vi "Header data_Cnsl.vi"(0 "base path":path=path "C:/", 5 "prompt (Create Folder)":string="logsConsole", 7 "file name":string, 11 "Error In":errorcluster) -> (4 "refnum out":refnum<file>, 15 "error out":errorcluster)   [LabVIEW 2018]
uses:
  Global_usbComm.vi
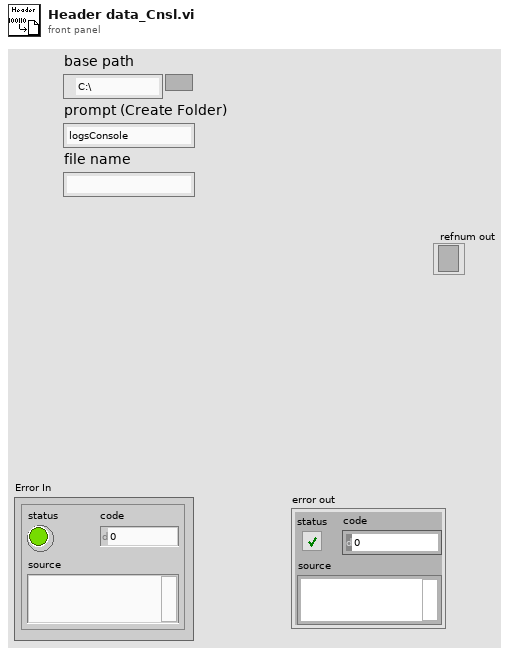
[diagram p1: front panel]
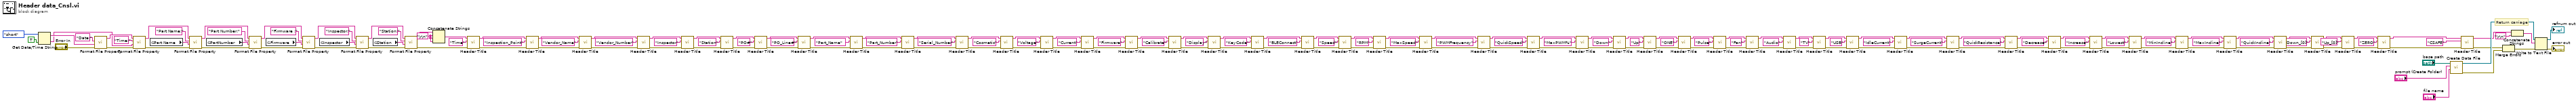
[diagram p0: block diagram]
diagram:
  w38 = "\r\n"
  # "Return carriage"
  n1 = Get Date/Time String(date format (0)=enum16{"short", "long", "abbreviated"}."short", want seconds? (F)=TRUE) -> (date string=w49:string, time string=w48:string)  [unwired: 1 in]
  n2 = call "Format File Property.vi"("Error In"="Error In", "File Property Value"=w49, "File Property Name"="Date:") -> ("Error Out"=w180:errorcluster, "String out"=w124:string)  [unwired: 7 in]
  n3 = call "Format File Property.vi"("Error In"=w180, "File Property Value"=w48, "File Property Name"="Time:", "String in"=w124) -> ("Error Out"=w41:errorcluster, "String out"=w42:string)  [unwired: 6 in]
  n4 = global read "Global_usbComm.vi" "Part Name"() -> (w112:string)
  n5 = call "Format File Property.vi"("Error In"=w41, "File Property Value"=w112, "File Property Name"="Part Name:", "String in"=w42) -> ("Error Out"=w175:errorcluster, "String out"=w122:string)  [unwired: 6 in]
  n6 = global read "Global_usbComm.vi" "PartNumber"() -> (w111:string)
  n7 = call "Format File Property.vi"("Error In"=w175, "File Property Value"=w111, "File Property Name"="Part Number:", "String in"=w122) -> ("Error Out"=w181:errorcluster, "String out"=w121:string)  [unwired: 6 in]
  n8 = global read "Global_usbComm.vi" "Firmware"() -> (w110:string)
  n9 = call "Format File Property.vi"("Error In"=w181, "File Property Value"=w110, "File Property Name"="Firmware :", "String in"=w121) -> ("Error Out"=w36:errorcluster, "String out"=w37:string)  [unwired: 6 in]
  n10 = global read "Global_usbComm.vi" "Inspector"() -> (w34:string)
  n11 = call "Format File Property.vi"("Error In"=w36, "File Property Value"=w34, "File Property Name"="Inspector:", "String in"=w37) -> ("Error Out"=w179:errorcluster, "String out"=w123:string)  [unwired: 6 in]
  n12 = global read "Global_usbComm.vi" "Station"() -> (w33:string)
  n13 = call "Format File Property.vi"("Error In"=w179, "File Property Value"=w33, "File Property Name"="Station:", "String in"=w123) -> ("Error Out"=w6:errorcluster, "String out"=w35:string)  [unwired: 6 in]
  n14 = Concatenate Strings(w35, w38, w38, w38) -> (w7:string)
  n15 = call "Header Title.vi"("Error In"=w6, "Header Title"="Time", "String in"=w7) -> ("Error Out"=w3:errorcluster, "String out"=w2:string)  [unwired: 7 in]
  n16 = call "Header Title.vi"("Error In"=w3, "Header Title"="Inspection_Point", "String in"=w2) -> ("Error Out"=w4:errorcluster, "String out"=w5:string)  [unwired: 7 in]
  n17 = call "Header Title.vi"("Error In"=w4, "Header Title"="Vendor_Name" ("File Property Name"), "String in"=w5) -> ("Error Out"=w23:errorcluster, "String out"=w31:string)  [unwired: 7 in]
  n18 = call "Header Title.vi"("Error In"=w23, "Header Title"="Vendor_Number" ("File Property Name"), "String in"=w31) -> ("Error Out"=w22:errorcluster, "String out"=w24:string)  [unwired: 7 in]
  n19 = call "Header Title.vi"("Error In"=w22, "Header Title"="Inspector" ("File Property Name"), "String in"=w24) -> ("Error Out"=w21:errorcluster, "String out"=w27:string)  [unwired: 7 in]
  n20 = call "Header Title.vi"("Error In"=w21, "Header Title"="Station" ("File Property Name"), "String in"=w27) -> ("Error Out"=w20:errorcluster, "String out"=w26:string)  [unwired: 7 in]
  n21 = call "Header Title.vi"("Error In"=w20, "Header Title"="PO#" ("File Property Name"), "String in"=w26) -> ("Error Out"=w14:errorcluster, "String out"=w13:string)  [unwired: 7 in]
  n22 = call "Header Title.vi"("Error In"=w14, "Header Title"="PO_Line#", "String in"=w13) -> ("Error Out"=w11:errorcluster, "String out"=w12:string)  [unwired: 7 in]
  n23 = call "Header Title.vi"("Error In"=w11, "Header Title"="Part_Name" ("File Property Name"), "String in"=w12) -> ("Error Out"=w16:errorcluster, "String out"=w18:string)  [unwired: 7 in]
  n24 = call "Header Title.vi"("Error In"=w16, "Header Title"="Part_Number" ("File Property Name"), "String in"=w18) -> ("Error Out"=w9:errorcluster, "String out"=w8:string)  [unwired: 7 in]
  n25 = call "Header Title.vi"("Error In"=w9, "Header Title"="Serial_Number" ("string"), "String in"=w8) -> ("Error Out"=w128:errorcluster, "String out"=w127:string)  [unwired: 7 in]
  n26 = call "Header Title.vi"("Error In"=w128, "Header Title"="Cosmetic", "String in"=w127) -> ("Error Out"=w132:errorcluster, "String out"=w131:string)  [unwired: 7 in]
  n27 = call "Header Title.vi"("Error In"=w132, "Header Title"="Voltage", "String in"=w131) -> ("Error Out"=w125:errorcluster, "String out"=w126:string)  [unwired: 7 in]
  n28 = call "Header Title.vi"("Error In"=w125, "Header Title"="Current" ("string"), "String in"=w126) -> ("Error Out"=w94:errorcluster, "String out"=w95:string)  [unwired: 7 in]
  n29 = call "Header Title.vi"("Error In"=w94, "Header Title"="Firmware" ("string"), "String in"=w95) -> ("Error Out"=w93:errorcluster, "String out"=w92:string)  [unwired: 7 in]
  n30 = call "Header Title.vi"("Error In"=w93, "Header Title"="Calibrate" ("string"), "String in"=w92) -> ("Error Out"=w137:errorcluster, "String out"=w158:string)  [unwired: 7 in]
  n31 = call "Header Title.vi"("Error In"=w137, "Header Title"="Display" ("string"), "String in"=w158) -> ("Error Out"=w69:errorcluster, "String out"=w68:string)  [unwired: 7 in]
  n32 = call "Header Title.vi"("Error In"=w69, "Header Title"="KeyCode", "String in"=w68) -> ("Error Out"=w70:errorcluster, "String out"=w67:string)  [unwired: 7 in]
  n33 = call "Header Title.vi"("Error In"=w70, "Header Title"="BLEConnect", "String in"=w67) -> ("Error Out"=w57:errorcluster, "String out"=w56:string)  [unwired: 7 in]
  n34 = call "Header Title.vi"("Error In"=w57, "Header Title"="Speed", "String in"=w56) -> ("Error Out"=w55:errorcluster, "String out"=w54:string)  [unwired: 7 in]
  n35 = call "Header Title.vi"("Error In"=w55, "Header Title"="RPM", "String in"=w54) -> ("Error Out"=w52:errorcluster, "String out"=w53:string)  [unwired: 7 in]
  n36 = call "Header Title.vi"("Error In"=w52, "Header Title"="MaxSpeed", "String in"=w53) -> ("Error Out"=w150:errorcluster, "String out"=w153:string)  [unwired: 7 in]
  n37 = call "Header Title.vi"("Error In"=w150, "Header Title"="PWMFrequency", "String in"=w153) -> ("Error Out"=w114:errorcluster, "String out"=w115:string)  [unwired: 7 in]
  n38 = call "Header Title.vi"("Error In"=w114, "Header Title"="QuickSpeed", "String in"=w115) -> ("Error Out"=w84:errorcluster, "String out"=w85:string)  [unwired: 7 in]
  n39 = call "Header Title.vi"("Error In"=w84, "Header Title"="MaxPWM%" ("Measured Data"), "String in"=w85) -> ("Error Out"=w136:errorcluster, "String out"=w157:string)  [unwired: 7 in]
  n40 = call "Header Title.vi"("Error In"=w136, "Header Title"="Down" ("Measured Data"), "String in"=w157) -> ("Error Out"=w133:errorcluster, "String out"=w134:string)  [unwired: 7 in]
  n41 = call "Header Title.vi"("Error In"=w133, "Header Title"="Up", "String in"=w134) -> ("Error Out"=w151:errorcluster, "String out"=w154:string)  [unwired: 7 in]
  n42 = call "Header Title.vi"("Error In"=w151, "Header Title"="ONE", "String in"=w154) -> ("Error Out"=w82:errorcluster, "String out"=w83:string)  [unwired: 7 in]
  n43 = call "Header Title.vi"("Error In"=w82, "Header Title"="Pulse", "String in"=w83) -> ("Error Out"=w149:errorcluster, "String out"=w152:string)  [unwired: 7 in]
  n44 = call "Header Title.vi"("Error In"=w149, "Header Title"="Fan", "String in"=w152) -> ("Error Out"=w116:errorcluster, "String out"=w117:string)  [unwired: 7 in]
  n45 = call "Header Title.vi"("Error In"=w116, "Header Title"="Audio", "String in"=w117) -> ("Error Out"=w119:errorcluster, "String out"=w120:string)  [unwired: 7 in]
  n46 = call "Header Title.vi"("Error In"=w119, "Header Title"="TV", "String in"=w120) -> ("Error Out"=w141:errorcluster, "String out"=w142:string)  [unwired: 7 in]
  n47 = call "Header Title.vi"("Error In"=w141, "Header Title"="USB", "String in"=w142) -> ("Error Out"=w89:errorcluster, "String out"=w88:string)  [unwired: 7 in]
  n48 = call "Header Title.vi"("Error In"=w89, "Header Title"="IdleCurrent" ("Measured Data"), "String in"=w88) -> ("Error Out"=w61:errorcluster, "String out"=w62:string)  [unwired: 7 in]
  n49 = call "Header Title.vi"("Error In"=w61, "Header Title"="SurgeCurrent", "String in"=w62) -> ("Error Out"=w60:errorcluster, "String out"=w59:string)  [unwired: 7 in]
  n50 = call "Header Title.vi"("Error In"=w60, "Header Title"="QuickResistance", "String in"=w59) -> ("Error Out"=w99:errorcluster, "String out"=w100:string)  [unwired: 7 in]
  n51 = call "Header Title.vi"("Error In"=w99, "Header Title"="Decrease", "String in"=w100) -> ("Error Out"=w86:errorcluster, "String out"=w87:string)  [unwired: 7 in]
  n52 = call "Header Title.vi"("Error In"=w86, "Header Title"="Increase" ("Measured Data"), "String in"=w87) -> ("Error Out"=w63:errorcluster, "String out"=w64:string)  [unwired: 7 in]
  n53 = call "Header Title.vi"("Error In"=w63, "Header Title"="Lowest", "String in"=w64) -> ("Error Out"=w44:errorcluster, "String out"=w45:string)  [unwired: 7 in]
  n54 = call "Header Title.vi"("Error In"=w44, "Header Title"="MinIncline", "String in"=w45) -> ("Error Out"=w47:errorcluster, "String out"=w46:string)  [unwired: 7 in]
  n55 = call "Header Title.vi"("Error In"=w47, "Header Title"="MaxIncline", "String in"=w46) -> ("Error Out"=w73:errorcluster, "String out"=w74:string)  [unwired: 7 in]
  n56 = call "Header Title.vi"("Error In"=w73, "Header Title"="QuickIncline" ("Measured Data"), "String in"=w74) -> ("Error Out"=w81:errorcluster, "String out"=w80:string)  [unwired: 7 in]
  n57 = call "Header Title.vi"("Error In"=w81, "Header Title"="Down_[0]", "String in"=w80) -> ("Error Out"=w77:errorcluster, "String out"=w76:string)  [unwired: 7 in]
  n58 = call "Header Title.vi"("Error In"=w77, "Header Title"="Up_[0]", "String in"=w76) -> ("Error Out"=w71:errorcluster, "String out"=w72:string)  [unwired: 7 in]
  n59 = call "Header Title.vi"("Error In"=w71, "Header Title"="ZERO", "String in"=w72) -> ("Error Out"=w90:errorcluster, "String out"=w91:string)  [unwired: 7 in]
  n60 = call "Create Data File.vi"("file name"="file name", "prompt (Create Folder)"="prompt (Create Folder)", "base path"="base path") -> ("Error Out"=w176:errorcluster, "File Refnum"=w178:refnum<file>)  [unwired: 7 in]
  n61 = call "Header Title.vi"("Error In"=w90, "Header Title"="CSAFE", "String in"=w91) -> ("Error Out"=w109:errorcluster, "String out"=w108:string)  [unwired: 7 in]
  n62 = Merge Errors(w109, w176) -> (w177:errorcluster)
  n63 = Concatenate Strings(w108, "\r\n") -> (w155:string)
  n64 = Write to Text File(file (use dialog)=w178, text=w155, error in=w177) -> (refnum out=→"refnum out":refnum<file>, error out=→"error out":errorcluster)  [unwired: 1 in, 1 out]
